vi "PoissonFit.vi"() -> ()   [LabVIEW 2014]
uses:
  <vilib>/gmath/SpecialFunctions.llb/Factorial.vi
  <vilib>/Waveform/WDTFileIO.llb/Read Waveform from File.vi
  <vilib>/Waveform/WDTOps.llb/WDT Get Final Time Value DBL.vi
  <vilib>/imath/engines/lvmath2/RunTimeEngine/Managers/WorkSpace/UID Generator.vi
  <vilib>/imath/engines/lvmath2/RunTimeEngine/BuiltInFunctions/size/NIMS_I32Row=size(GRow).vi
  <instcachedir>/0/NIMS_I32Row=size(GRow)_E5C05C6B13124B29B774CC4F993D3C59.lvgen/NIMS_I32Row=size(GRow)_E5C05C6B13124B29B774CC4F993D3C59_000.vi
  <vilib>/imath/engines/lvmath2/RunTimeEngine/RunTimeType/NIMS_RunTimeType_From StrictType (excl LVString).vi
  <instcachedir>/0/NIMS_RunTimeType_From StrictType (excl LVString)_15A5391EEA9C4AACB9955AC755B83D29.lvgen/NIMS_RunTimeType_From StrictType (excl LVString)_15A5391EEA9C4AACB9955AC755B83D29_000.vi
  <vilib>/imath/engines/lvmath2/RunTimeEngine/LocalVariableDefStatement/MC_LocalVariableDefStatement_Display.vi
  <vilib>/imath/engines/lvmath2/RunTimeEngine/IndexRead/NIMS M(S,S).vi
  <instcachedir>/0/NIMS M(S,S)_AC51E74150A542F7991B9634C66F3096.lvgen/NIMS M(S,S)_AC51E74150A542F7991B9634C66F3096_002.vi
  <vilib>/imathl/engines/lvmath/Functions/Error Handling/Create Error.vi
  <vilib>/imath/engines/lvmath2/RunTimeEngine/BuiltInFunctions/max/1 input/NIMS_max(RV).vi
  <instcachedir>/0/NIMS_max(RV)_237633DB1D604D5BA7001287DF3C7957.lvgen/NIMS_max(RV)_237633DB1D604D5BA7001287DF3C7957_000.vi
  <vilib>/imath/engines/lvmath2/RunTimeEngine/BuiltInFunctions/min/1 input/NIMS_min(RV).vi
  <instcachedir>/0/NIMS_min(RV)_EE2DD3E2888846108C5160A664B67832.lvgen/NIMS_min(RV)_EE2DD3E2888846108C5160A664B67832_000.vi
  <vilib>/imath/engines/lvmath2/RunTimeEngine/RangeToken/NIMS_Range.vi
  <instcachedir>/0/NIMS_Range_9BCE657718DF4976A877346C61F22738.lvgen/NIMS_Range_9BCE657718DF4976A877346C61F22738_000.vi
  <vilib>/imath/engines/lvmath2/RunTimeEngine/RangeToken/NIMS_Range_R3 - Integer.vi
  <instcachedir>/0/NIMS_Range_R3 - Integer_66B9031982364693905FDE422E56E490.lvgen/NIMS_Range_R3 - Integer_66B9031982364693905FDE422E56E490_000.vi
  <vilib>/imath/engines/lvmath2/RunTimeEngine/CommandStatement/MC_CommandStatement_break.vi
  <instcachedir>/0/NIMS M(S,S)_AC51E74150A542F7991B9634C66F3096.lvgen/NIMS M(S,S)_AC51E74150A542F7991B9634C66F3096_000.vi
  <vilib>/imath/engines/lvmath2/RunTimeEngine/ErrorHandling/NIMS_Create Error From Enums.vi
  <vilib>/imath/engines/lvmath2/RunTimeEngine/ArithmeticOperatorToken/NIMS_ArithmeticOperator_power(S).vi
  <instcachedir>/0/NIMS_ArithmeticOperator_power(S)_CAFE680B12A64A3A8F5E28A20C679B7D.lvgen/NIMS_ArithmeticOperator_power(S)_CAFE680B12A64A3A8F5E28A20C679B7D_017.vi
  <vilib>/imath/engines/lvmath2/RunTimeEngine/ArithmeticOperatorToken/NIMS_ArithmeticOperator_rightdiv(C,C).vi
  <instcachedir>/0/NIMS_ArithmeticOperator_rightdiv(C,C)_B4CE00C486B54A9B9073334614CFE190.lvgen/NIMS_ArithmeticOperator_rightdiv(C,C)_B4CE00C486B54A9B9073334614CFE190_000.vi
  <vilib>/imath/engines/lvmath2/RunTimeEngine/Managers/SymbolTable/Clear UID.vi
  <vilib>/imath/engines/lvmath2/RunTimeEngine/NodeEndStatement/NIMS_NodeEndStatement_Output.vi
  <instcachedir>/0/NIMS_NodeEndStatement_Output_53EC0D466D134D7ABD903AC30B43404B.lvgen/NIMS_NodeEndStatement_Output_53EC0D466D134D7ABD903AC30B43404B_005.vi
  <instcachedir>/0/NIMS_NodeEndStatement_Output_53EC0D466D134D7ABD903AC30B43404B.lvgen/NIMS_NodeEndStatement_Output_53EC0D466D134D7ABD903AC30B43404B_000.vi
  <vilib>/imath/engines/lvmath2/RunTimeEngine/ErrorHandling/NIMS_Finalize Error.vi
  <vilib>/Analysis/NI_AALBase.lvlib
  <vilib>/gmath/NI_Gmath.lvlib
  <vilib>/imath/engines/lvmath2/RunTimeEngine/Managers/SymbolTable/NIMS_WorkSpace.lvlib
panel:
  in  "Histogram Intervals":i32=10
  out "Poisson Fit":cluster{"k":dbl[], "out":dbl[]}[](graph)=[{"k"=[15.5, 18.5, 21.5, 24.5, 27.5, 30.5, 33.5, 36.5, 39.5, 42.5], "out"=[16.0, 39.0, 64.0, 82.0, 49.0, 33.0, 11.0, 3.0, 2.0, 1.0]}, {"k"=[15.0, 16.0, 17.0, 18.0, 19.0, 20.0, 21.0, 22.0, 23.0, 24.0, 25.0, 26.0, 27.0, 28.0, 29.0, 30.0, 31.0, 32.0, 33.0, 34.0, 35.0, 36.0, 37.0, 38.0, 39.0, 40.0, 41.0, 42.0, 43.0], "out"=[9.290618088558686, 14.144966039830624, 20.268904278251444, 27.430583789900332, 35.168895848524656, 42.8357151435031, 49.689429566463325, 55.01975019268403, 58.27309194320805, 59.14718832235627, 57.633020301304036, 53.99770671306802, 48.71793094556812, 42.38459992264374, 35.6030639350208, 28.909687915236933, 22.717419277908807, 17.293635425308107, 12.765847241227458, 9.146354082244159, 6.365862441241944, 4.307566918573724, 2.836008922606881, 1.818030983018519, 1.1355701217008, 0.6915622041157883, 0.4108891534697715, 0.23831570901246446, 0.13500862026845875]}]
  in  "Data File":path=path "C:/Users/cnee1/Desktop/week8/constant"
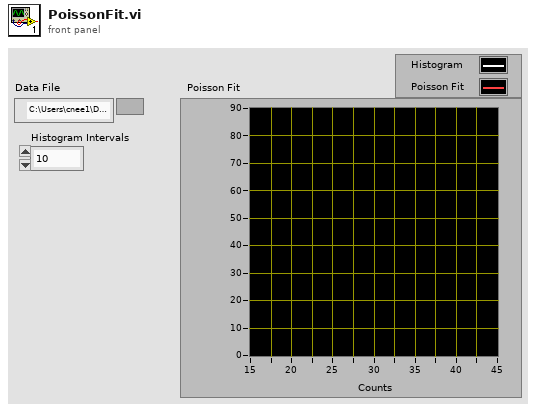
[diagram p1: front panel]
types:
  T1 = cluster{"X Values":dbl[], "Histogram: h(x)":i32[]}
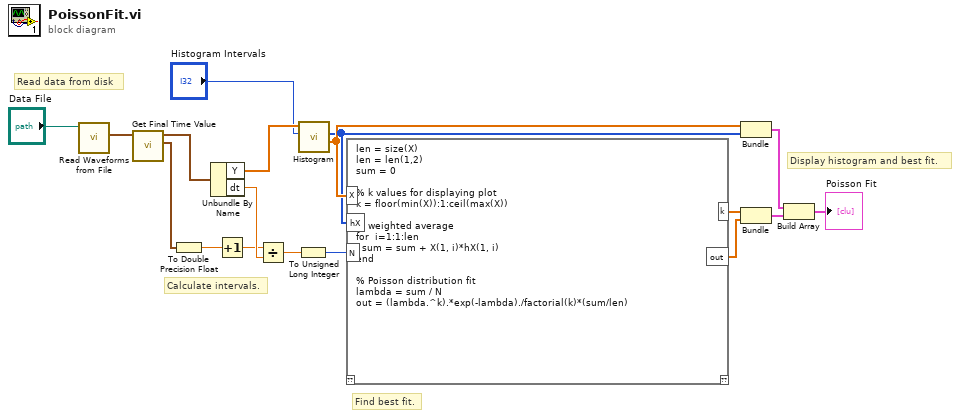
[diagram p0: block diagram]
diagram:
  # "Find best fit."
  # "Display histogram and best fit."
  # "Calculate intervals."
  # "Read data from disk"
  n1 = call-poly <vilib>:"Read Waveforms from File.vi"("file path (dialog if empty)"="Data File") -> ("first waveform in record"=w5:waveform(dbl))  [unwired: 5 in, 3 out]
  n2 = call-poly <vilib>:"Get Final Time Value.vi"("waveform in"=w5) -> ("tf"=w15:timestamp, "waveform out"=w16:waveform(dbl))  [unwired: 8 in, 1 out]
  n3 = To Double Precision Float(number=w15) -> (double precision float=w14:dbl)
  n4 = Unbundle By Name(w16) -> ("Y"=w17:dbl[], "dt"=w13:dbl)
  n5 = Increment(x=w14) -> (x+1=w11:dbl)
  n6 = Divide(x=w11, y=w13) -> (x/y=w12:dbl)
  n7 = To Unsigned Long Integer(number=w12) -> (unsigned 32bit integer=w6:u32)
  n8 = call <vilib>:"Histogram.vi"("intervals"="Histogram Intervals", "X"=w17) -> ("X Values"=w10:dbl[], "Histogram: h(x)"=w9:i32[])  [unwired: 6 in, 2 out]
  n9 = mathscript code="len = size(X)\nlen = len(1,2)\nsum = 0\n\n% k values for displaying plot\nk = floor(min(X)):1:ceil(max(X))\n\n% weighted average\nfor  i=1:1:len\n  sum = sum + X(1, i)*hX(1, i)\nend\n\n% Poisson distribution fit\nlambda = sum / N\nout = (lambda.^k).*exp(-lambda)./factorial(k)*(sum/len)"("X"=w10, "hX"=w9, "N"=w6) -> ("out"=w8:cdb[], "k"=w4:dbl[])  [unwired: 1 in, 1 out]
  n10 = Bundle("X Values"=w10, "Histogram: h(x)"=w9) -> (w3:T1)  [unwired: 1 in]
  n11 = Bundle("k"=w4, "out"=w8) -> (w2:cluster{"k":dbl[], "out":cdb[]})  [unwired: 1 in]
  n12 = Build Array(w3, w2) -> (→"Poisson Fit":cluster{"k":dbl[], "out":cdb[]}[])
